vi "SysDef.CreateSection.vi"(7 "GUID (Default Section)":string="03D3BB89-1485-13A6-56005DE6430FF8B7", 8 "error in (no error)":errorcluster, 10 "Name":string, 11 "nodeID":u64) -> (0 "error out":errorcluster, 1 "New NodeID":u64, 2 "newItem":bool, 3 "nodeID out":u64)   [LabVIEW 2015, in "Advanced System Definition.lvlib"]
uses:
  Advanced System Definition.lvlib
  NationalInstruments.VeriStand.SystemDefinitionAPI
  <vilib>/NI Veristand/Custom Device API/Custom Device API.lvlib
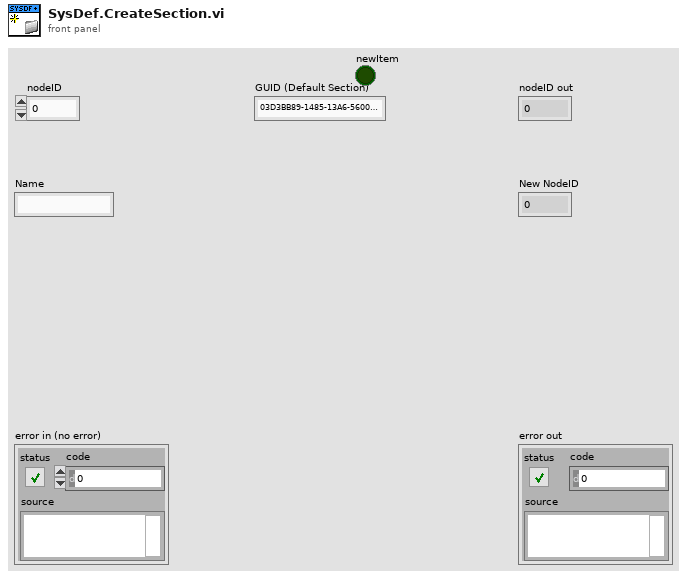
[diagram p1: front panel]
types:
  T1 = typedef "Custom Device API.lvlib/Custom Device Item Ref.ctl" = u64
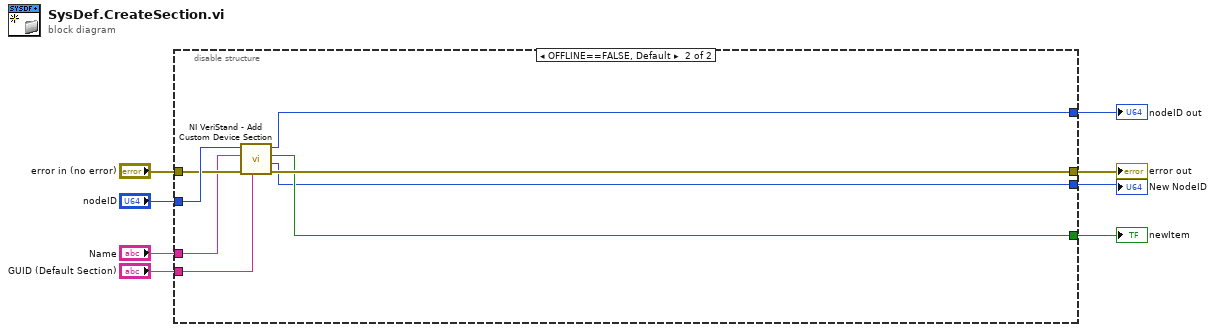
[diagram p0: block diagram]
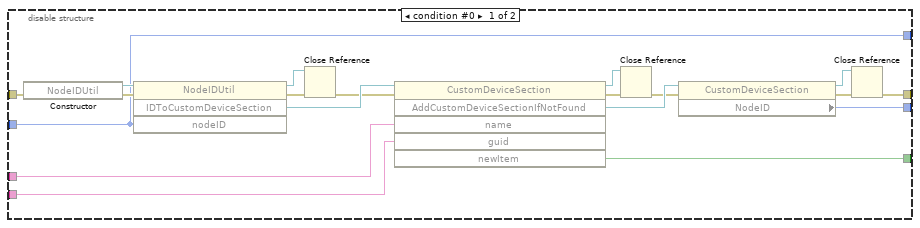
[diagram p2: hidden frame]
diagram:
  n1 = disable-structure shown="OFFLINE==FALSE, Default" {
    disable-tunnel: "nodeID" -> [w9 w35]
    disable-tunnel: "error in (no error)" -> [w24 w34]
    disable-tunnel: "Name" -> [w16 w32]
    disable-tunnel: "GUID (Default Section)" -> [w15 w33]
    disable-tunnel: [w12 w31] -> w4
    disable-tunnel: [w11 w29] -> w3
    disable-tunnel: [w10 w30] -> w2
    disable-tunnel: [w9 w28] -> w1
    frame condition #0 {
      n2 = constructor class="NodeIDUtil"(error in=w24) -> (reference out=w26:refnum<k24>, error out=w25:errorcluster)  [unwired: 2 in, 1 out]
      n3 = invoke class="NodeIDUtil" method="IDToCustomDeviceSection"(reference=w26, error in=w25, "nodeID"=w9) -> (reference out=w23:refnum<k24>, error out=w14:errorcluster, "IDToCustomDeviceSection"=w27:refnum<k24>)  [unwired: 1 in, 1 out]
      n4 = Close Reference(reference=w23, error in (no error)=w14) -> (error out=w13:errorcluster)
      n5 = invoke class="CustomDeviceSection" method="AddCustomDeviceSectionIfNotFound"(reference=w27, error in=w13, "name"=w16, "guid"=w15) -> (reference out=w21:refnum<k24>, error out=w22:errorcluster, "AddCustomDeviceSectionIfNotFound"=w20:refnum<k24>, "newItem"=w10:bool)  [unwired: 2 in, 2 out]
      n6 = Close Reference(reference=w21, error in (no error)=w22) -> (error out=w19:errorcluster)
      n7 = property class="CustomDeviceSection"(reference=w20, error in=w19) -> (reference out=w18:refnum<k24>, error out=w17:errorcluster, "NodeID"=w11:u64)
      n8 = Close Reference(reference=w18, error in (no error)=w17) -> (error out=w12:errorcluster)
    }
    frame condition #1 (active) {
      n9 = call <vilib>:"NI VeriStand - Add Custom Device Section.vi"("GUID (Default Section)"=w33, "error in (no error)"=w34, "Section Name"=w32, "Parent Ref in"=w35) -> ("error out"=w31:errorcluster, "Section Ptr"=w29:T1, "Newly Created?"=w30:bool, "Parent Ref out"=w28:T1)  [unwired: 4 in]
    }
  }
  "New NodeID" <- w3
  "nodeID out" <- w1
  "error out" <- w4
  "newItem" <- w2
